vi "getTaskReference.vi"(8 "error in (no error)":errorcluster, 11 "ExampleTask_MsgUserEventStopNotifier In":refnum<class "ExampleTask_MsgUserEventStopNotifier.lvclass">) -> (0 "error out":errorcluster, 2 "taskRef":refnum<vi>, 3 "ExampleTask_MsgUserEventStopNotifier Out":refnum<class "ExampleTask_MsgUserEventStopNotifier.lvclass">)   [LabVIEW 2023, in "ExampleTask_MsgUserEventStopNotifier.lvclass"]
doc: "Returns the VI reference related to the task to handle."
uses:
  ExampleTask_MsgUserEventStopNotifier.lvclass
  myTask.vi
  ExampleTask_MsgUserEventStopNotifier.lvclass/ExampleTask_MsgUserEventStopNotifier.ctl
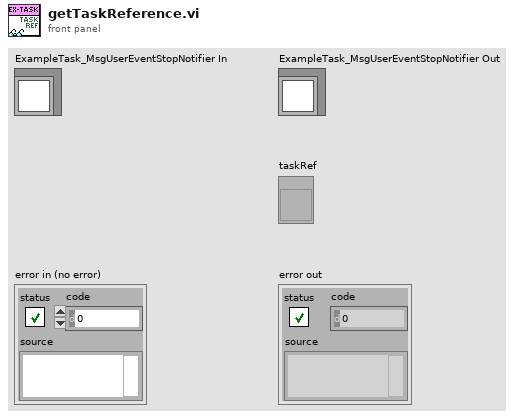
[diagram p1: front panel]
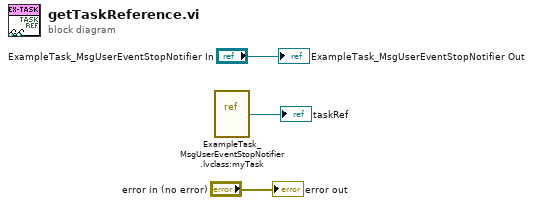
[diagram p0: block diagram]
diagram:
  n1 = vi-ref "ExampleTask_MsgUserEventStopNotifier.lvclass:myTask.vi"() -> (→"taskRef":refnum<vi>)
  "error out" <- "error in (no error)"
  "ExampleTask_MsgUserEventStopNotifier Out" <- "ExampleTask_MsgUserEventStopNotifier In"
